vi "Configure ISIM IMPU.vi"(8 "error in (no error)":errorcluster, 9 "IMPUs":string[](array[string]), 10 "SIM Profile Name (\"\")":string, 11 "VISA resource name":refnum<visa-resource-name>) -> (0 "error out":errorcluster, 3 "VISA resource name out":refnum<visa-resource-name>)   [LabVIEW 2015, in "Rohde&Schwarz CMXP Base.lvlib"]
doc: "Specifies the IP multimedia public identities (IMPUs)\n\nAttribute:\nRSCMXPBASE_ATTR_ISIM_IP_MULTIMEDIA_PUBLIC_IDENTITIES\n\nRemote-control command:\n[CONFigure:]SIMProfile:ISIM:IMPU"
uses:
  <instrlib>/Rohde&Schwarz CMXP Base/Rohde&Schwarz CMXP Base.lvlib
  <instrlib>/Rohde&Schwarz CMXP Base/Private/rsidr_core.llb/rsidr_core.lvlib
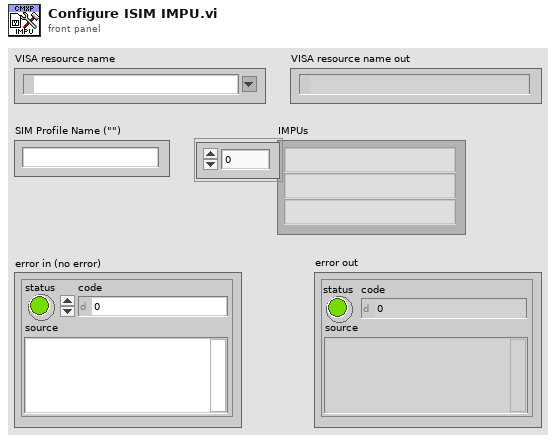
[diagram p1: front panel]
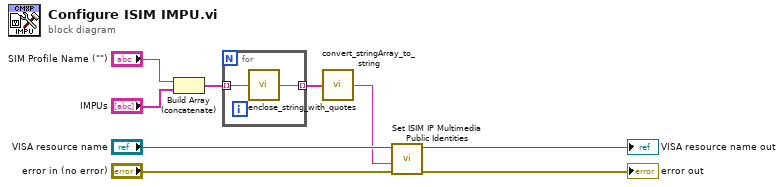
[diagram p0: block diagram]
diagram:
  n1 = Build Array (concatenate)("SIM Profile Name (\"\")", "IMPUs") -> (w3:string[])
  n2 = for {
    tunnel: w3 -> [w11] mode=indexing
    tunnel: [w10] -> w2 mode=indexing
    n3 = call <instrlib>:"enclose_string_with_quotes.vi"("String to enclose"=w11) -> ("String out"=w10:string)  [unwired: 4 in]
  }
  n4 = call <instrlib>:"convert_stringArray_to_string.vi"("string array in"=w2) -> ("string out"=w1:string)  [unwired: 4 in]
  n5 = call "Set ISIM IP Multimedia Public Identities"("error in (no error)"="error in (no error)", "ISIM IP Multimedia Public Identities ()"=w1, "instrument handle"="VISA resource name") -> ("error out"=→"error out":errorcluster, "instrument handle out"=→"VISA resource name out":refnum<visa-resource-name>)  [unwired: 7 in]
